vi "3.13 x 3.13 Complex Multiplication.vi"(6 "input valid":bool, 8 "conjugate B":bool=TRUE, 9 "B":T1, 10 "conjugate A":bool=TRUE, 11 "A":T1) -> (0 "output valid":bool, 1 "product":T2)   [LabVIEW 2020]
uses:
  <vilib>/rvi/FXPMathLib/FxpInterpret/XNode/nifxpmath_Interpret.xnode
panel:
  out "Imag 2":fxp<+/-,18,18>
  out "Real 2":fxp<+/-,18,18>
  out "Imag":fxp<+/-,25,25>
  out "Real":fxp<+/-,25,25>
types:
  T1 = cluster{"Real":fxp<+/-,16,3>, "Imag":fxp<+/-,16,3>}
  T2 = cluster{"Real":fxp<+/-,33,7>, "Imag":fxp<+/-,33,7>}
  T3 = cluster{"Real":fxp<+/-,25,25>, "Imag":fxp<+/-,25,25>}
  T4 = cluster{"Real":fxp<+/-,18,18>, "Imag":fxp<+/-,18,18>}
  T5 = cluster{"Real":fxp<+/-,48,48>, "Imag":fxp<+/-,48,48>}
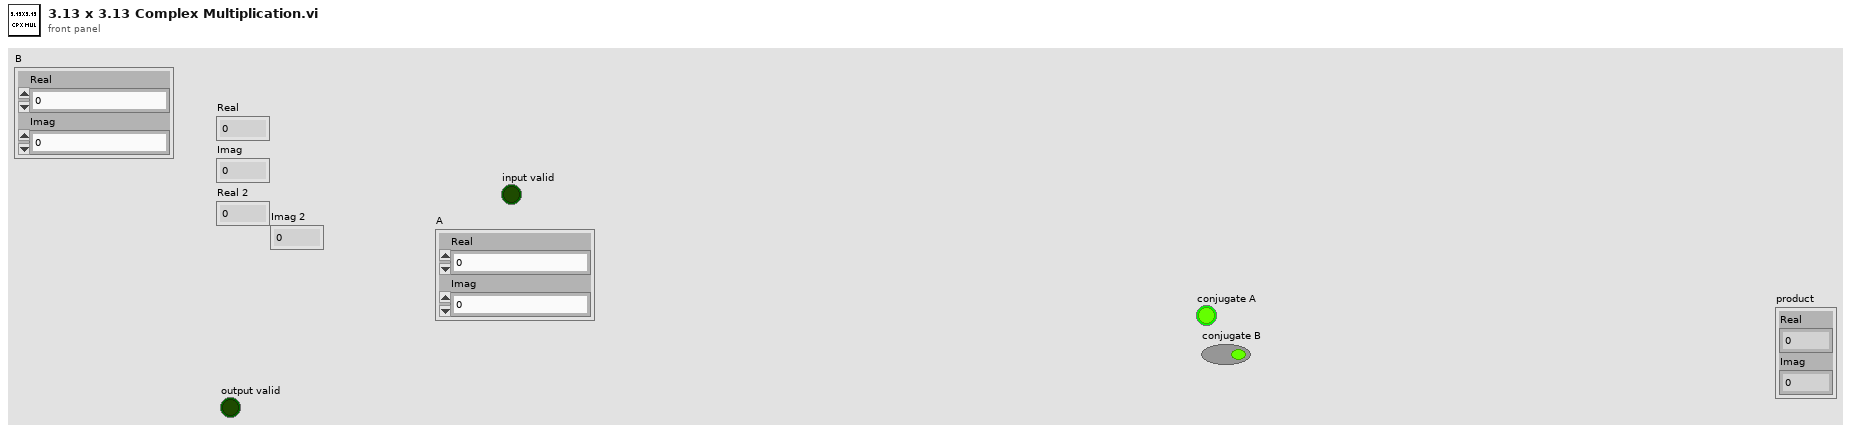
[diagram p1: front panel]
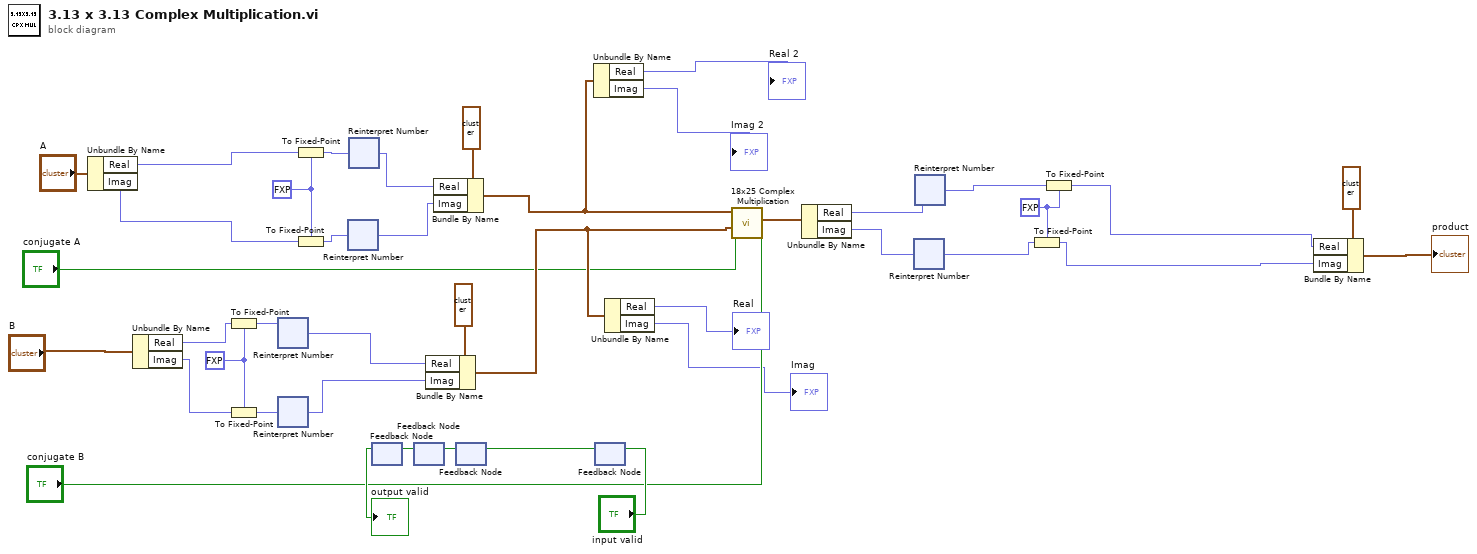
[diagram p0: block diagram]
diagram:
  w9 = fxp<+/-,25,12> 0.0 ("fixed-point type")
  w26 = fxp<+/-,18,5> 0.0 ("fixed-point type")
  w30 = fxp<+/-,33,7> 0.0 ("fixed-point type")
  n1 = Unbundle By Name("A") -> ("Real"=w23:fxp<+/-,16,3>, "Imag"=w22:fxp<+/-,16,3>)
  n2 = Unbundle By Name("B") -> ("Real"=w8:fxp<+/-,16,3>, "Imag"=w7:fxp<+/-,16,3>)
  n3 = To Fixed-Point(fixed-point type=w9, number=w8) -> (fixed-point=w6:fxp<+/-,25,12>)
  n4 = To Fixed-Point(fixed-point type=w9, number=w7) -> (fixed-point=w5:fxp<+/-,25,12>)
  n5 = xnode "Reinterpret Number"("x"=w6) -> ("y"=w19:fxp<+/-,25,25>)
  n6 = xnode "Reinterpret Number"("x"=w5) -> ("y"=w18:fxp<+/-,25,25>)
  n7 = To Fixed-Point(fixed-point type=w26, number=w23) -> (fixed-point=w25:fxp<+/-,18,5>)
  n8 = To Fixed-Point(fixed-point type=w26, number=w22) -> (fixed-point=w24:fxp<+/-,18,5>)
  n9 = xnode "Reinterpret Number"("x"=w24) -> ("y"=w20:fxp<+/-,18,18>)
  n10 = xnode "Reinterpret Number"("x"=w25) -> ("y"=w21:fxp<+/-,18,18>)
  n11 = feedback #1() -> (→"output valid":bool)  [unwired: 1 in]
  n12 = feedback #2() -> (w36:bool)  [unwired: 1 in]
  n13 = feedback-in #1(w36) -> ()
  n14 = Bundle By Name(cluster=T3 {"Real"=0.0, "Imag"=0.0} ("Complex"), "Real"=w19, "Imag"=w18) -> (w12:T3)
  n15 = Bundle By Name(cluster=T4 {"Real"=0.0, "Imag"=0.0} ("Complex"), "Real"=w21, "Imag"=w20) -> (w15:T4)
  n16 = feedback #3() -> (w35:bool)  [unwired: 1 in]
  n17 = feedback-in #2(w35) -> ()
  n18 = Unbundle By Name(w15) -> ("Real"=→"Real 2":fxp<+/-,18,18>, "Imag"=→"Imag 2":fxp<+/-,18,18>)
  n19 = feedback #4() -> (w10:bool)  [unwired: 1 in]
  n20 = feedback-in #3(w10) -> ()
  n21 = feedback-in #4("input valid") -> ()
  n22 = Unbundle By Name(w12) -> ("Real"=→"Real":fxp<+/-,25,25>, "Imag"=→"Imag":fxp<+/-,25,25>)
  n23 = call "18x25 Complex Multiplication.vi"("conjugate B"="conjugate B", "B"=w12, "conjugate A"="conjugate A", "A"=w15) -> ("product"=w33:T5)  [unwired: 7 in]
  n24 = Unbundle By Name(w33) -> ("Real"=w32:fxp<+/-,48,48>, "Imag"=w31:fxp<+/-,48,48>)
  n25 = xnode "Reinterpret Number"("x"=w31) -> ("y"=w28:fxp<+/-,48,22>)
  n26 = xnode "Reinterpret Number"("x"=w32) -> ("y"=w29:fxp<+/-,48,22>)
  n27 = To Fixed-Point(fixed-point type=w30, number=w28) -> (fixed-point=w3:fxp<+/-,33,7>)
  n28 = To Fixed-Point(fixed-point type=w30, number=w29) -> (fixed-point=w4:fxp<+/-,33,7>)
  n29 = Bundle By Name(cluster=T2 {"Real"=0.0, "Imag"=0.0} ("Complex"), "Real"=w4, "Imag"=w3) -> (→"product":T2)
